vi "add_ElementOfPastAgents.vi"(0 "MoAgSy_Host":refnum<class "MoAgSy_Host.lvclass">, 3 "Cluster":cluster{"Agent ID":string, "Destination":string}, 5 "error in (no error)":errorcluster) -> (14 "dup MoAgSy_Host":refnum<class "MoAgSy_Host.lvclass">, 19 "error out":errorcluster)   [LabVIEW 2009, in "MoAgSy.lvlib" / "MoAgSy_Host.lvclass"]
doc: "<B>protected</B> VI removes agent id from running agents list and add agent destination and id to past agents cluster of mobile agent host class.\nIs called by public remove agent VI\n\nF.Berck@gsi.de\nGSI Darmstadt 2009"
uses:
  MoAgSy_Host.lvclass
  MoAgSy_Host.lvclass/MoAgSy_Host.ctl
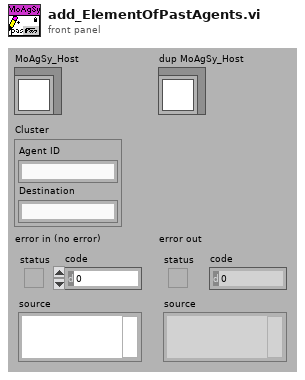
[diagram p1: front panel]
types:
  T1 = cluster{"Agent ID":string, "Destination":string}[]
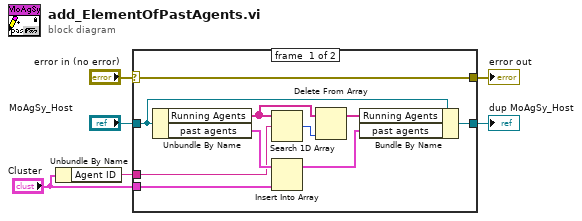
[diagram p0: block diagram]
diagram:
  n1 = Unbundle By Name("Cluster") -> ("Agent ID"=w1:string)
  n2 = case shown="No Error" "error in (no error)" {
    selector: "error in (no error)" -> [w16 w17]
    tunnel: [w16 w17] -> w5
    tunnel: [w15 w18] -> w3
    tunnel: "MoAgSy_Host" -> [w14 w18]
    tunnel: "Cluster" -> [w11 _]
    tunnel: w1 -> [w10 _]
    frame #0 {
      n3 = Unbundle By Name(w14) -> ("Running Agents"=w9:string[], "past agents"=w13:T1)
      n4 = Search 1D Array(1D array=w9, element=w10) -> (index of element=w8:i32)  [unwired: 1 out]
      n5 = Insert Into Array(array=w13, new element=w11) -> (w12:T1)  [unwired: 1 in]
      n6 = Delete From Array(array=w9, index=w8) -> (array with subset deleted=w7:string[])  [unwired: 1 in, 1 out]
      n7 = Bundle By Name(cluster=w14, "Running Agents"=w7, "past agents"=w12) -> (w15:refnum<class "MoAgSy_Host.lvclass">)
    }
    frame #1 {
    }
  }
  "error out" <- w5
  "dup MoAgSy_Host" <- w3
